vi "knob-2020.vi"() -> ()   [LabVIEW 2020]
panel:
  out "?":dbl
  in  "Temperature":dbl(knob) scale=0.0..100.0
  in  "?":bool
  in  "VISA resource name":refnum<visa-resource-name>
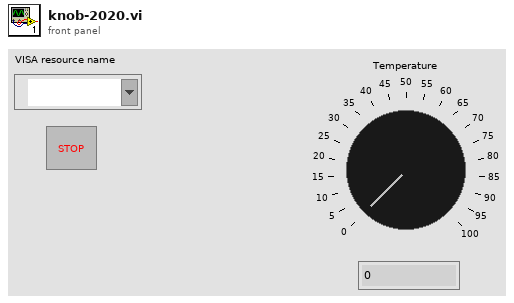
[diagram p1: front panel]
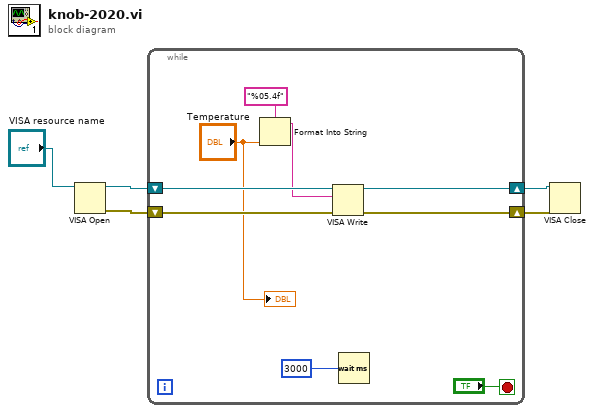
[diagram p0: block diagram]
diagram:
  n1 = VISA Open(VISA resource name="VISA resource name") -> (VISA resource name=w5:refnum<visa-resource-name>, error out=w4:errorcluster)  [unwired: 4 in]
  n2 = while {
    shift-right: [w11] -> w2
    shift-left: w5 -> [w14]
    shift-right: [w12] -> w3
    shift-left: w4 -> [w13]
    stop <- "?" stop-if-true
    n3 = Format Into String(format string="%05.4f", "Temperature") -> (resulting string=w8:string)  [unwired: 2 in, 1 out]
    n4 = VISA Write(VISA resource name=w14, write buffer=w8, error in (no error)=w13) -> (VISA resource name out=w11:refnum<visa-resource-name>, error out=w12:errorcluster)  [unwired: 1 out]
    n5 = Wait (ms)(milliseconds to wait=u32 3000) -> ()  [unwired: 1 out]
    "?" <- "Temperature"
  }
  n6 = VISA Close(VISA resource name=w2, error in (no error)=w3) -> ()  [unwired: 1 out]
